vi "Unflatten Header.vi"(8 "error in":errorcluster, 10 "Flattened Data in":u8[](array[numeric])=[0, 0, 0, 0, 0, 0, 0, 0, 0, 0, 0, 0, 0, 0, 0, 0, 0, 0, 0, 0, 0, 0, 0, 0, 0, 0, 0, 0, 0, 0, 0, 0], 11 "Header in":T1) -> (0 "error out":errorcluster, 2 "Flatten Data out":u8[](array[numeric]), 3 "Header out":T1)   [LabVIEW 2021, in "ChannelCommon.lvlib"]
uses:
  ChannelCommon.lvlib
  typedef/FIFO Header.ctl
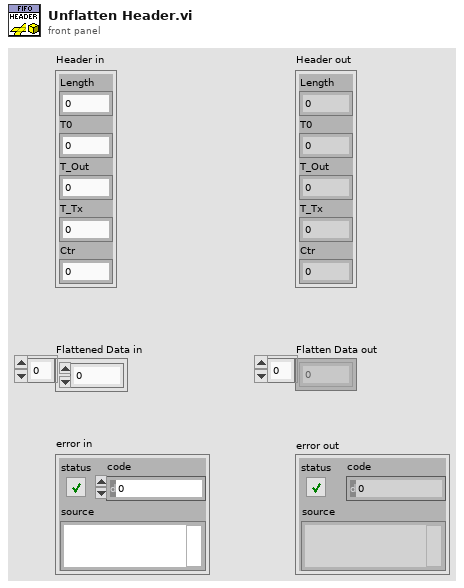
[diagram p1: front panel]
types:
  T1 = typedef "ChannelCommon.lvlib/FIFO Header.ctl" = cluster{"Length":u64, "T0":u64, "T_Out":u64, "T_Tx":u64, "Ctr":u64}
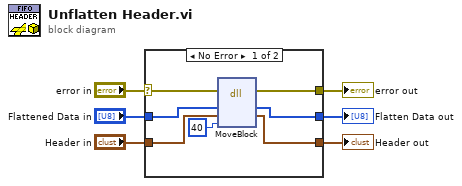
[diagram p0: block diagram]
diagram:
  n1 = case shown="No Error" "error in" {
    selector: "error in" -> [w7 w16]
    tunnel: "Header in" -> [w13 w14]
    tunnel: "Flattened Data in" -> [w12 w15]
    tunnel: [w11 w16] -> w4
    tunnel: [w10 w14] -> w3
    tunnel: [w9 w15] -> w2
    frame No Error {
      n2 = dll-call lib="LabVIEW" fn="MoveBlock"(error in=w7, "source"=w12, "dest"=w13, "size"=u64 40) -> (error out=w11:errorcluster, "source"=w9:u8[], "dest"=w10:T1)  [unwired: 4 in, 1 out]
    }
    frame Error {
    }
  }
  "Header out" <- w3
  "error out" <- w4
  "Flatten Data out" <- w2
